vi "Utility Create Data Directory.vi"(3 "Folder Name":string) -> (1 "Path":path)   [LabVIEW 2015]
doc: "Creates folder in default data directory. If the folder already exists, it does nothing."
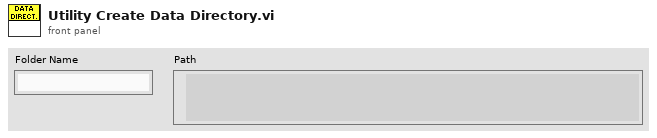
[diagram p1: front panel]
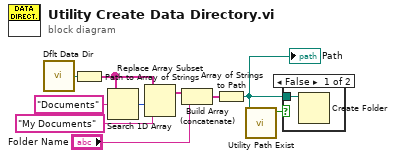
[diagram p0: block diagram]
diagram:
  n1 = call <vilib>:"Dflt Data Dir.vi"() -> ("App:Default Data Directory"=w10:path)
  n2 = Path to Array of Strings(0:w10) -> (2:w4:string[])  [unwired: 1 out]
  n3 = Search 1D Array(1D array=w4, element="Documents") -> (index of element=w8:i32)  [unwired: 1 in]
  n4 = Replace Array Subset(array=w4, new element="My Documents" ("element"), index=w8) -> (w7:string[])
  n5 = Build Array (concatenate)(w7, "Folder Name") -> (w6:string[])
  n6 = Array of Strings to Path(0:w6) -> (2:w1:path)  [unwired: 1 in]
  "Path" <- w1
  n7 = call "Utility Path Exist.vi"("Path"=w1) -> ("Exists?"=w3:bool)  [unwired: 10 in]
  n8 = case shown="False" w3 {
    tunnel: w1 -> [w11 _]
    frame False {
      n9 = Create Folder(path (use dialog)=w11) -> ()  [unwired: 2 in, 3 out]
    }
    frame True {
    }
  }
